vi "get_temporary_file_path.vi"(8 "error in (no error)":errorcluster, 11 "Image.lvclass in":refnum<class "Image.lvclass">) -> (0 "error out":errorcluster, 2 "temporary file path":path, 3 "Image.lvclass out":refnum<class "Image.lvclass">)   [LabVIEW 2010, in "Image.lvclass"]
uses:
  Image.lvclass
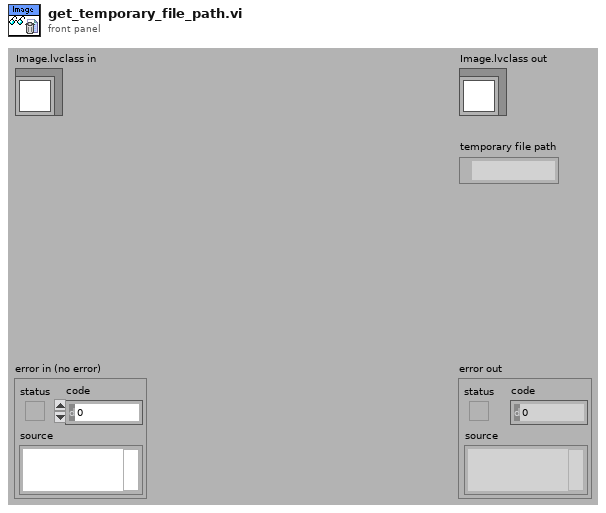
[diagram p1: front panel]
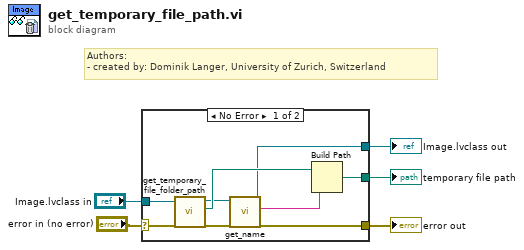
[diagram p0: block diagram]
diagram:
  # "Authors: \n- created by: Dominik Langer, University of Zurich, Switzerland"
  n1 = case shown="No Error" "error in (no error)" {
    selector: "error in (no error)" -> [w14 w15]
    tunnel: [w11 w15] -> w4
    tunnel: [w8 w16] -> w2
    tunnel: "Image.lvclass in" -> [w9 w16]
    tunnel: [w6 _] -> w1
    frame No Error {
      n2 = call-dynamic "get_temporary_file_folder_path.vi"("error in (no error)"=w14, "Image in"=w9) -> ("error out"=w12:errorcluster, "temp file folder"=w13:path, "Image out"=w10:refnum<class "Image.lvclass">)  [unwired: 7 out]
      n3 = call-dynamic "get_name.vi"("error in (no error)"=w12, "Image in"=w10) -> ("error out"=w11:errorcluster, "name"=w7:string, "Image out"=w8:refnum<class "Image.lvclass">)  [unwired: 7 out]
      n4 = Build Path(base path=w13, name or relative path=w7) -> (appended path=w6:path)
    }
    frame Error {
    }
  }
  "error out" <- w4
  "Image.lvclass out" <- w2
  "temporary file path" <- w1
